vi "Database-GetComponent.vi"(8 "error in":errorcluster, 9 "Serial component":string, 10 "Ref component":string, 11 "Idx":i32) -> (0 "error out":errorcluster, 1 "Serial product":string, 2 "Ref product":string)   [LabVIEW 2016]
doc: "Go to DB->WriteStationValues action\nReturn boolean flag to show if data was saved to DB successfully\n\nWabco 2017 All right reserved\nAuthor: maciej.szupienko@wabco-auto.com"
uses:
  Database.Action.ctl
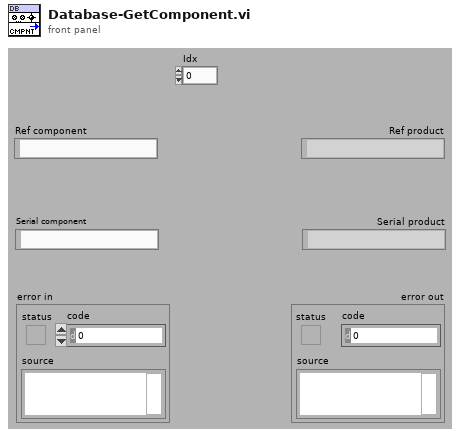
[diagram p1: front panel]
types:
  T1 = typedef "Database.Action.ctl" = enum32{"idle", "constructor", "destructor", "--- DB ---", "Setup", "Disconnect", "Connect", "GetAllStatuses"}
  T2 = cluster{"Ref component":string, "Serial component":string}
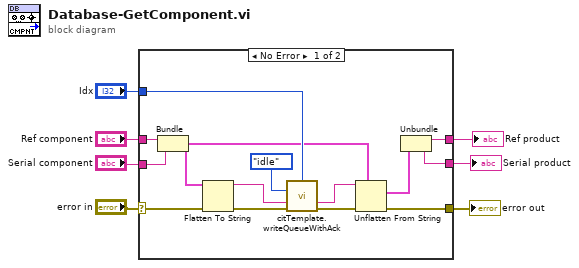
[diagram p0: block diagram]
diagram:
  n1 = case shown="No Error" "error in" {
    selector: "error in" -> [w19 w24]
    tunnel: [w17 w24] -> w6
    tunnel: "Idx" -> [w21 _]
    tunnel: "Serial component" -> [w8 w22]
    tunnel: "Ref component" -> [w15 w23]
    tunnel: [w10 w23] -> w2
    tunnel: [w9 w22] -> w1
    frame No Error {
      n2 = Bundle("Ref component"=w15, "Serial component"=w8) -> (w12:T2)  [unwired: 1 in]
      n3 = Flatten To String(anything=w12, error in (no error)=w19) -> (data string=w13:string, error out=w18:errorcluster)  [unwired: 2 in, 1 out]
      n4 = call "citTemplate.writeQueueWithAck.vi"("instance (0)"=w21, "event in"=Database.Action."idle" ("Action"), "(flatten) data in"=w13, "error in (no error)"=w18) -> ("notification data"=w16:string, "error out"=w20:errorcluster)  [unwired: 9 in, 1 out]
      n5 = Unflatten From String(type=w12, binary string=w16, error in (no error)=w20) -> (value=w11:T2, error out=w17:errorcluster)  [unwired: 2 in, 1 out]
      n6 = Unbundle(w11) -> ("Ref component"=w10:string, "Serial component"=w9:string)
    }
    frame Error {
    }
  }
  "error out" <- w6
  "Serial product" <- w1
  "Ref product" <- w2
